vi "SpeedDistanceM1M2.vi"(4 "Distance2":u32 max=127 step=1, 5 "Speed2":i32 max=127 step=1, 6 "Immediate":u8 max=127 step=1, 7 "Distance1":u32 max=127 step=1, 8 "error in (no error)":errorcluster, 9 "Address":u8, 10 "Speed1":i32 max=127 step=1, 11 "VISA Refnum in":refnum<visa-resource-name>) -> (0 "error out":errorcluster, 2 "Valid":bool, 3 "VISA Refnum out":refnum<visa-resource-name>)   [LabVIEW 2015, in "Ion Motion Roboclaw.lvlib"]
uses:
  <instrlib>/Ion Motion Roboclaw/Ion Motion Roboclaw.lvlib
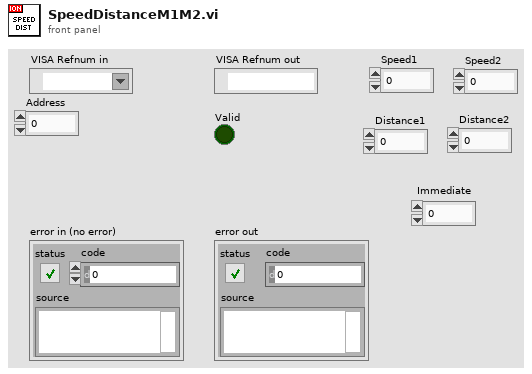
[diagram p1: front panel]
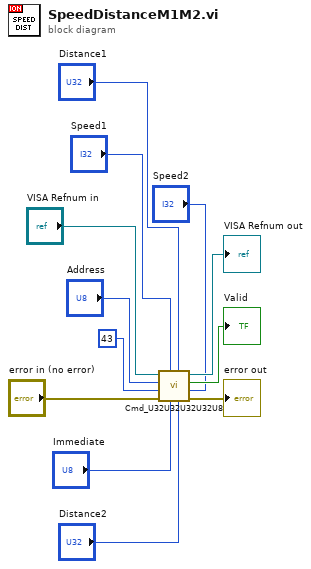
[diagram p0: block diagram]
diagram:
  n1 = call <instrlib>:"Cmd_U32U32U32U32U8.vi"("Arg3"="Speed2", "Arg4"="Distance2", "Arg2"="Distance1", "Arg5"="Immediate", "Arg1"="Speed1", "error in (no error)"="error in (no error)", "Cmd"=u8 43, "Address"="Address", "VISA Refnum in"="VISA Refnum in") -> ("error out"=→"error out":errorcluster, "Valid"=→"Valid":bool, "VISA Refnum out"=→"VISA Refnum out":refnum<visa-resource-name>)
